vi "user32_CloseWindow.vi"(0 "hWnd":u32, 11 "错误输入（无错误）":errorcluster) -> (4 "dup hWnd":u32, 6 "success?":bool, 15 "错误输出":errorcluster)   [LabVIEW 2011]
doc: "该函数最小化指定的窗口，但并不销毁该窗口。"
uses:
  user32.dll
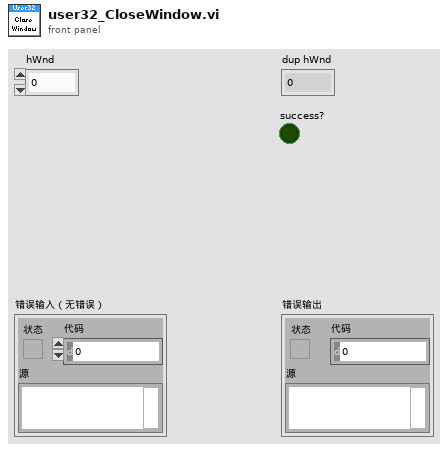
[diagram p1: front panel]
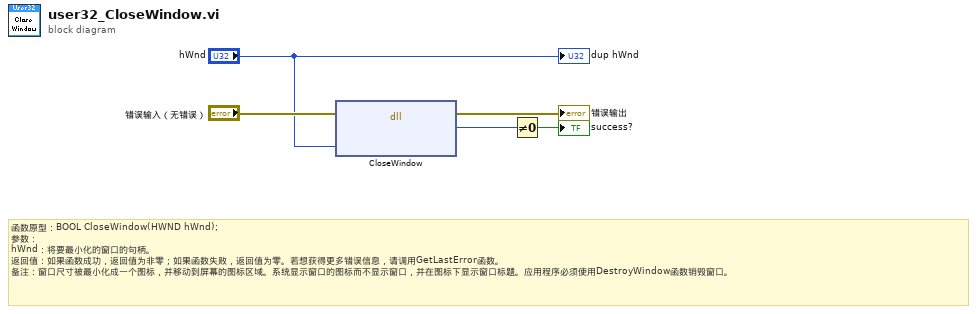
[diagram p0: block diagram]
diagram:
  # "函数原型：BOOL CloseWindow(HWND hWnd);\n参数：\nhWnd：将要最小化的窗口的句柄。\n返回值：如果函数成功，返回值为非零；如果函数失败，返回值为零。若想获得更多错误信息，请调用GetLastError函数。\n备注：窗口尺寸被最小化成一个图标，并移动到屏幕的图标区域。系统显示窗口的图标而不显示窗口，并在图标下显示窗口标题。应用程序必须使用DestroyWindow函数销毁窗口。"
  n1 = dll-call lib="user32.dll" fn="CloseWindow"(error in="错误输入（无错误）", "hWnd"="hWnd") -> (error out=→"错误输出":errorcluster, "Bool"=w2:u8)  [unwired: 3 in, 1 out]
  n2 = Not Equal To 0?(x=w2) -> (x != 0?=→"success?":bool)
  "dup hWnd" <- "hWnd"
